vi "Finalize.vi"(8 "error in":errorcluster, 11 "logging execution unit in":refnum<class "Logging Execution Unit.lvclass">) -> (0 "error out":errorcluster, 3 "logging execution unit out":refnum<class "Logging Execution Unit.lvclass">)   [LabVIEW 2020, in "Ballard MIL-STD-1553 Engine.lvlib" / "Implementation.lvlib" / "Logging Execution Unit.lvclass"]
uses:
  Logging Execution Unit.lvclass
  C:/Users/nitest/Desktop/Git 2020/niveristand-aim-milStd1553-custom-device/Source/Custom Device Support/Engine/Implementation/Execution Unit/Execution Unit.lvclass
  Execution Unit/Execution Unit.lvclass/Execution Unit.ctl
  Execution Unit/Execution Unit.lvclass
  <instrlib>/BTICardLib/BTICardLV.lvlib
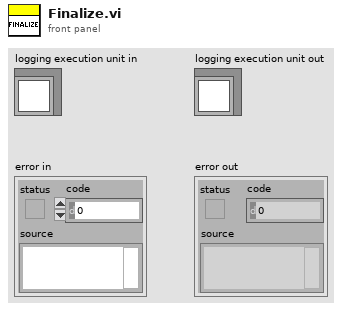
[diagram p1: front panel]
types:
  T1 = typedef "Ballard MIL-STD-1553 Engine.lvlib/Custom Device.lvlib/Hardware Handles.ctl" = cluster{"core handle":u64, "core reader handle":u64, "channel handles":u64[]}
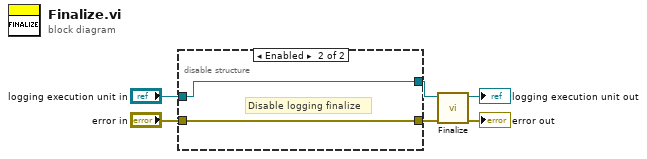
[diagram p0: block diagram]
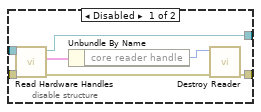
[diagram p2: hidden frame]
diagram:
  n1 = disable-structure shown="Enabled" {
    disable-tunnel: [w13 w14] -> w4
    disable-tunnel: "error in" -> [w12 w14]
    disable-tunnel: "logging execution unit in" -> [w11 w15]
    disable-tunnel: [w7 w15] -> w1
    frame Disabled {
      n2 = call "Read Hardware Handles.vi"("error in"=w12, "Execution Unit in"=w11) -> ("error out"=w8:errorcluster, "hardware handles"=w10:T1, "Execution Unit out"=w7:refnum<class "Logging Execution Unit.lvclass">)  [unwired: 7 in]
      n3 = Unbundle By Name(w10) -> ("core reader handle"=w9:u64)
      n4 = call <instrlib>:"Destroy Reader.vi"("error in (no error)"=w8, "reader handle in"=w9) -> ("error out"=w13:errorcluster)  [unwired: 9 in]
    }
    frame Enabled {
      # "Disable logging finalize"
    }
  }
  n5 = call-parent "Finalize.vi"("error in (no error)"=w4, "Execution Unit Implementation in"=w1) -> ("error out"=→"error out":errorcluster, "Execution Unit Implementation out"=→"logging execution unit out":refnum<class "Logging Execution Unit.lvclass">)  [unwired: 8 in]
